vi "Init DAQmx Lock-in.vi"(0 "DAQmx Device Name":tag="Dev1", 1 "Amplitude":dbl=0.04 format="%#_6pV", 5 "Desired frequency":dbl=96.0 format="%#_6pHz", 7 "Input channel":string="ai0", 9 "Input range":dbl=1.0 format="%#_6pV", 11 "error in":errorcluster) -> (3 "Samples per read":i32, 4 "CO task out":refnum<k21>, 6 "AO task out":refnum<k21>, 10 "AI task out":refnum<k21>, 12 "Actual clock":dbl=961538.4615384615 format="%#_10p", 14 "Lockin parameters":T1={"Frequency"=0.0, "Phase"=0.0, "Syncronous"=FALSE, "Points per sine wave"=0, "DDS"=FALSE, "Frequency word"=0, "Phase word"=0, "DDS modulus"=15120, "DDS clock"=125000000.0} {"DDS clock" format="%_17pHz"; "DDS modulus" format="0x%x (%d)"; "Phase" format="%#_gdeg"; "Frequency" format="%_17pHz"}, 15 "error out":errorcluster)   [LabVIEW 2021]
uses:
  SoftwareLockin/Lockin Parameters.ctl
  <vilib>/DAQmx/create/channels.llb/DAQmx Create Channel (CO-Pulse Generation-Frequency).vi
  <vilib>/DAQmx/configure/timing.llb/DAQmx Timing (Sample Clock).vi
  <vilib>/DAQmx/miscellaneous.llb/DAQmx Fill In Error Info.vi
  <vilib>/DAQmx/create/channels.llb/DAQmx Create Channel (AI-Voltage-Basic).vi
  <vilib>/DAQmx/configure/timing.llb/DAQmx Timing (Implicit).vi
  <vilib>/DAQmx/create/channels.llb/DAQmx Create Channel (AO-Voltage-Basic).vi
  <vilib>/DAQmx/write.llb/DAQmx Write (Analog 1D DBL 1Chan NSamp).vi
  <resource>/objmgr/daqmx.rc
  <vilib>/Analysis/NI_AALBase.lvlib
panel:
  in  "Desired update time":dbl=0.1 format="%#_6ps"
  in  "Desired clock":dbl=2000000.0 format="%#_13pHz"
  out "Waveform Graph":dbl[](graph)
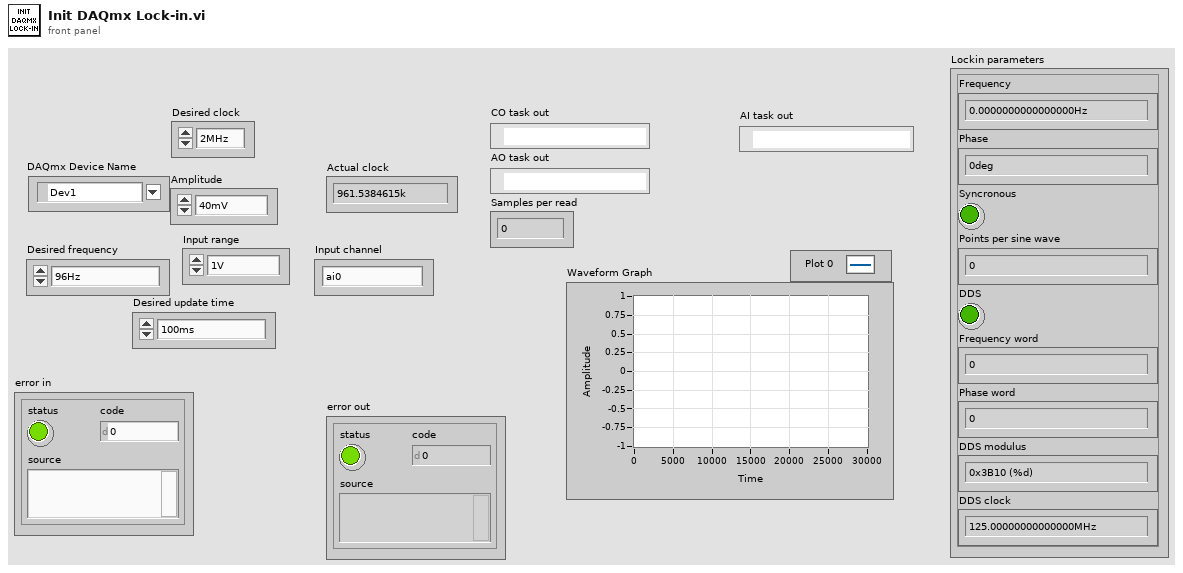
[diagram p1: front panel]
types:
  T1 = typedef "Lockin Parameters.ctl" = cluster{"Frequency":dbl, "Phase":dbl, "Syncronous":bool, "Points per sine wave":i32, "DDS":bool, "Frequency word":u32, "Phase word":u32, "DDS modulus":i64, "DDS clock":dbl}
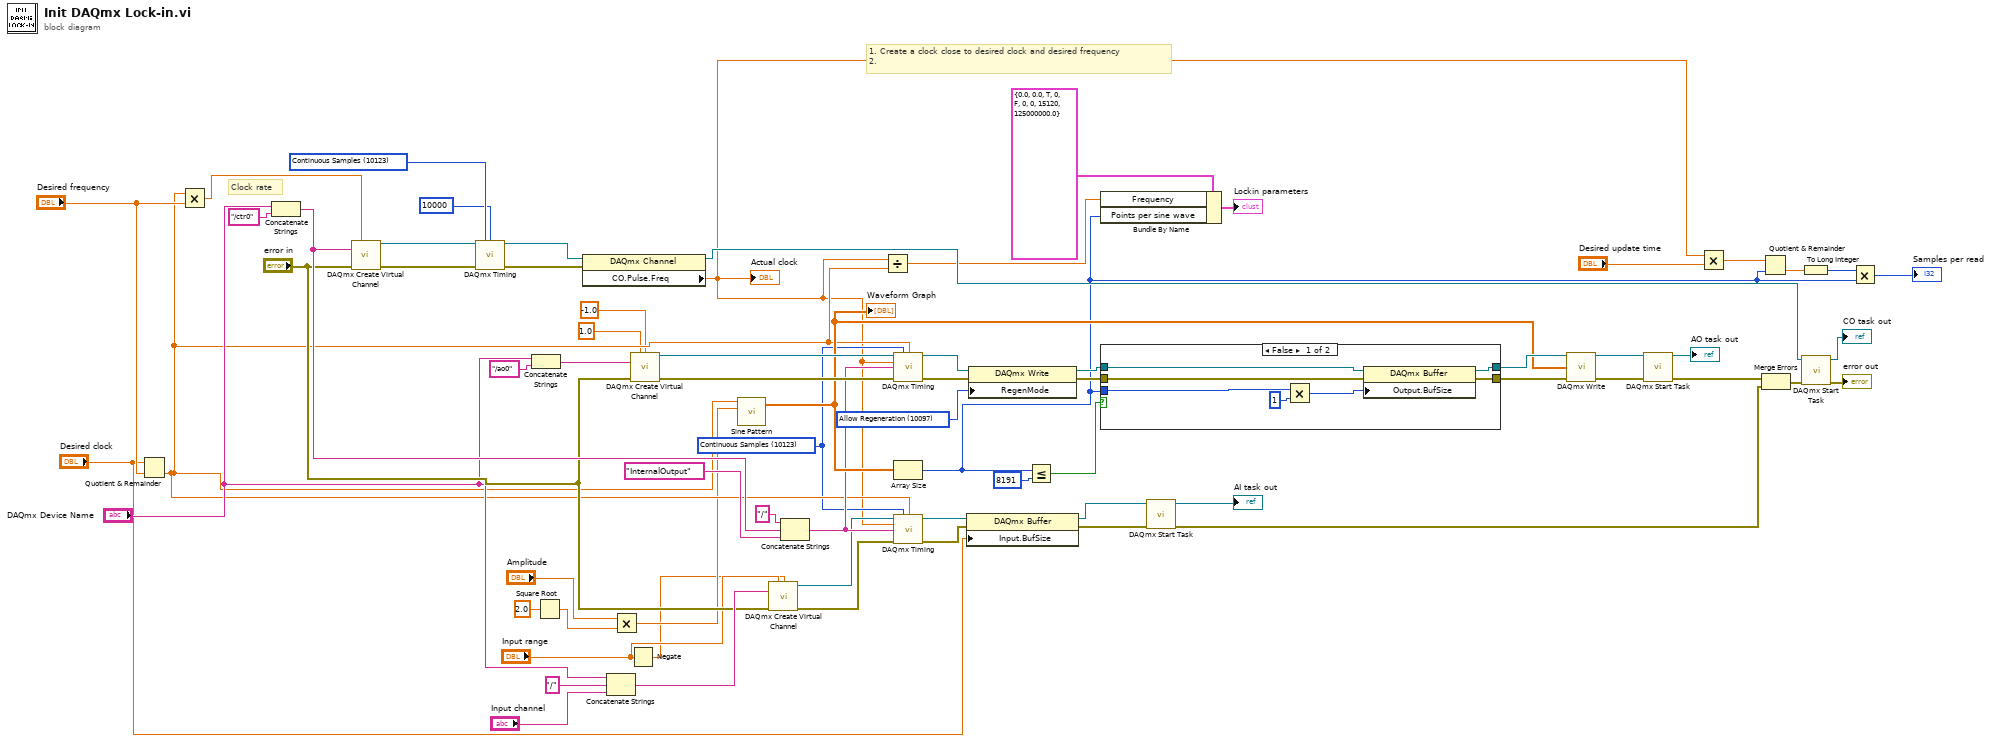
[diagram p0: block diagram]
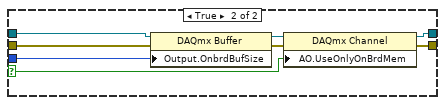
[diagram p2: hidden frame]
diagram:
  w32 = 10123 items=["Finite Samples"=10178, "Continuous Samples"=10123, "Hardware Timed Single Point"=12522] ("sample mode")
  w50 = 10097 items=["Allow Regeneration"=10097, "Do Not Allow Regeneration"=10158] ("RegenMode")
  w66 = 10123 items=["Finite Samples"=10178, "Continuous Samples"=10123, "Hardware Timed Single Point"=12522] ("sample mode")
  # "1. Create a clock close to desired clock and desired frequency\n2."
  # "Clock rate"
  n1 = Quotient & Remainder(x="Desired clock", y="Desired frequency") -> (floor(x/y)=w33:dbl)  [unwired: 1 out]
  n2 = Multiply(x=w33, y="Desired frequency") -> (x*y=w67:dbl)
  n3 = Concatenate Strings("DAQmx Device Name", "/ctr0") -> (w53:string)
  n4 = call-poly <vilib>:"DAQmx Create Virtual Channel.vi"("frequency"=w67, "counter"=w53, "error in"="error in") -> ("task out"=w65:refnum<k21>, "error out"=w64:errorcluster)  [unwired: 11 in]
  n5 = call-poly <vilib>:"DAQmx Timing.vi"("task/channels in"=w65, "sample mode"=w66, "samples per channel"=10000, "error in"=w64) -> ("task out"=w63:refnum<k21>, "error out"=w62:errorcluster)  [unwired: 10 in]
  n6 = Concatenate Strings("DAQmx Device Name", "/ao0") -> (w56:string)
  n7 = Square Root(x=2.0) -> (sqrt(x)=w8:dbl)
  n8 = property class="DAQmx Channel"(reference=w63, error in=w62) -> (reference out=w61:refnum<k21>, "CO.Pulse.Freq"=w18:dbl)  [unwired: 1 out]
  "Actual clock" <- w18
  n9 = Concatenate Strings("DAQmx Device Name", "/", "Input channel") -> (w37:string)
  n10 = Multiply(x="Amplitude", y=w8) -> (x*y=w6:dbl)
  n11 = Negate(x="Input range") -> (-x=w2:dbl)
  n12 = call-poly <vilib>:"DAQmx Create Virtual Channel.vi"("maximum value"=1.0, "minimum value"=-1.0, "physical channels"=w56, "error in"="error in") -> ("task out"=w58:refnum<k21>, "error out"=w59:errorcluster)  [unwired: 10 in]
  n13 = call <vilib>:"Sine Pattern.vi"("amplitude"=w6, "samples"=w33) -> ("Sinusoidal Pattern"=w41:dbl[])  [unwired: 2 in, 1 out]
  "Waveform Graph" <- w41
  n14 = call-poly <vilib>:"DAQmx Create Virtual Channel.vi"("maximum value"="Input range", "minimum value"=w2, "physical channels"=w37, "error in"="error in") -> ("task out"=w21:refnum<k21>, "error out"=w20:errorcluster)  [unwired: 10 in]
  n15 = Concatenate Strings("/", w53, "InternalOutput" ("string")) -> (w34:string)
  n16 = Divide(x=w18, y=w33) -> (x/y=w11:dbl)
  n17 = call-poly <vilib>:"DAQmx Timing.vi"("task/channels in"=w58, "sample mode"=w32, "samples per channel"=w33, "rate"=w18, "source"=w34, "error in"=w59) -> ("task out"=w52:refnum<k21>, "error out"=w51:errorcluster)  [unwired: 8 in]
  n18 = Array Size(array=w41) -> (size(s)=w10:i32)
  n19 = call-poly <vilib>:"DAQmx Timing.vi"("task/channels in"=w21, "sample mode"=w32, "samples per channel"=w33, "rate"=w18, "source"=w34, "error in"=w20) -> ("task out"=w31:refnum<k21>, "error out"=w30:errorcluster)  [unwired: 8 in]
  n20 = property class="DAQmx Buffer"(reference=w31, error in=w30, "Input.BufSize"="Desired clock") -> (reference out=w25:refnum<k21>, error out=w26:errorcluster)
  n21 = property class="DAQmx Write"(reference=w52, error in=w51, "RegenMode"=w50) -> (reference out=w43:refnum<k21>, error out=w42:errorcluster)
  n22 = Less Or Equal?(x=w10, y=8191) -> (x <= y?=w39:bool)
  n23 = Bundle By Name(cluster=T1 {"Frequency"=0.0, "Phase"=0.0, "Syncronous"=TRUE, "Points per sine wave"=0, "DDS"=FALSE, "Frequency word"=0, "Phase word"=0, "DDS modulus"=15120, "DDS clock"=125000000.0} ("Lockin parameters"), "Frequency"=w11, "Points per sine wave"=w10) -> (→"Lockin parameters":T1)
  n24 = case shown="False" w39 {
    selector: w39 -> [_ w77]
    tunnel: [w73 w84] -> w45
    tunnel: [w74 w83] -> w44
    tunnel: w43 -> [w76 w82]
    tunnel: w42 -> [w75 w80]
    tunnel: w10 -> [w71 w78]
    frame False {
      n25 = Multiply(x=w71, y=1) -> (x*y=w70:i32)
      n26 = property class="DAQmx Buffer"(reference=w76, error in=w75, "Output.BufSize"=w70) -> (reference out=w73:refnum<k21>, error out=w74:errorcluster)
    }
    frame True {
      n27 = property class="DAQmx Buffer"(reference=w82, error in=w80, "Output.OnbrdBufSize"=w78) -> (reference out=w81:refnum<k21>, error out=w79:errorcluster)
      n28 = property class="DAQmx Channel"(reference=w81, error in=w79, "AO.UseOnlyOnBrdMem"=w77) -> (reference out=w84:refnum<k21>, error out=w83:errorcluster)
    }
  }
  n29 = call <vilib>:"DAQmx Start Task.vi"("task/channels in"=w25, "error in"=w26) -> ("task out"=→"AI task out":refnum<k21>, "error out"=w24:errorcluster)  [unwired: 12 in]
  n30 = call-poly <vilib>:"DAQmx Write.vi"("task/channels in"=w45, "data"=w41, "error in"=w44) -> ("task out"=w48:refnum<k21>, "error out"=w49:errorcluster)  [unwired: 10 in, 1 out]
  n31 = call <vilib>:"DAQmx Start Task.vi"("task/channels in"=w48, "error in"=w49) -> ("task out"=→"AO task out":refnum<k21>, "error out"=w27:errorcluster)  [unwired: 12 in]
  n32 = Multiply(x=w18, y="Desired update time") -> (x*y=w17:dbl)
  n33 = Quotient & Remainder(x=w17, y=w10) -> (floor(x/y)=w16:dbl)  [unwired: 1 out]
  n34 = Merge Errors(w27, w24) -> (w28:errorcluster)
  n35 = To Long Integer(number=w16) -> (32bit integer=w14:i32)
  n36 = call <vilib>:"DAQmx Start Task.vi"("task/channels in"=w61, "error in"=w28) -> ("task out"=→"CO task out":refnum<k21>, "error out"=→"error out":errorcluster)  [unwired: 12 in]
  n37 = Multiply(x=w14, y=w10) -> (x*y=→"Samples per read":i32)
